vi "Parameter Druckregler.vi"(0 "Regelparameter":sgl[][](array[numeric]), 1 "Werte PMA":sgl[](array[numeric]), 2 "Werte FT-IR":sgl[](array[numeric]), 3 "Werte Ausgang":sgl[](array[numeric]), 4 "Werte NDIR":sgl[](array[numeric]), 5 "Werte Durchfluss":sgl[](array[numeric]), 6 "Werte Gaskühler":sgl[](array[numeric]), 7 "Werte Filterblock":sgl[](array[numeric]), 8 "Werte Kalter Block":sgl[](array[numeric]), 9 "Aktionen":T1) -> (10 "Werte Kalter Block":sgl[](array[numeric]), 12 "Werte Gaskühler":sgl[](array[numeric]), 13 "Werte Filterblock":sgl[](array[numeric]), 14 "Regleparameter":sgl[][](array[numeric]), 15 "Werte PMA":sgl[](array[numeric]), 16 "Werte FT-IR":sgl[](array[numeric]), 17 "Werte Ausgang":sgl[](array[numeric]), 18 "Werte NDIR":sgl[](array[numeric]), 19 "Werte Durchfluss":sgl[](array[numeric]))   [LabVIEW 2020, in "Regler.lvlib" / "Druckregler.lvlib"]
uses:
  Druckregler.lvlib
  Aktionen Param. Druckregler.ctl
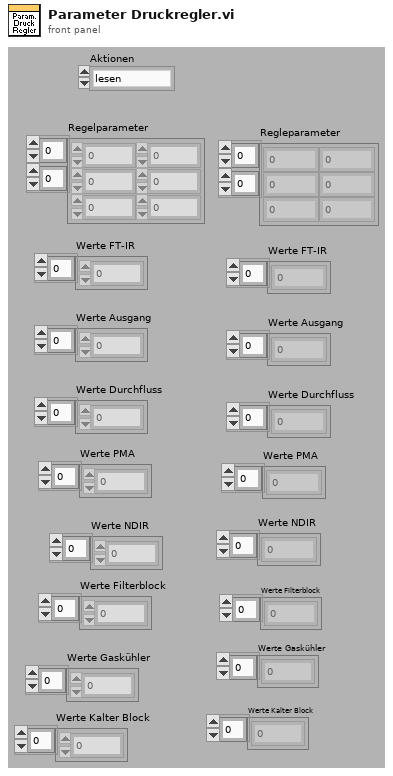
[diagram p1: front panel]
types:
  T1 = typedef "Regler.lvlib/Druckregler.lvlib/Aktionen Param. Druckregler.ctl" = enum16{"lesen", "schreiben", "Regler FT-IR", "Regler Ausgang", "Regler Durchfluss", "Regler PMA", "Regler NDIR", "Regler Filterblock", "Regler Gaskühler", "Regler Kalter Block"}
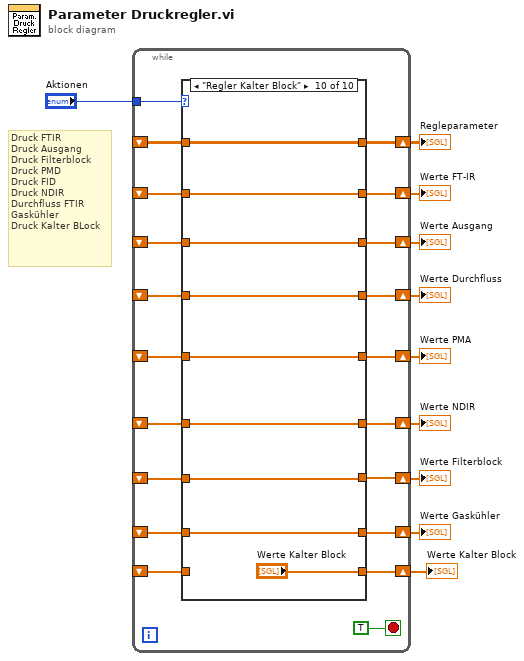
[diagram p0: block diagram]
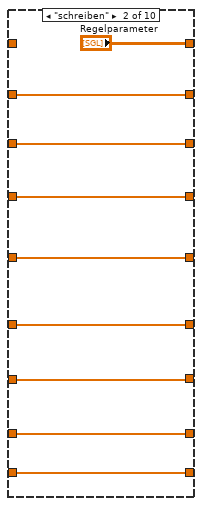
[diagram p3: hidden frame]
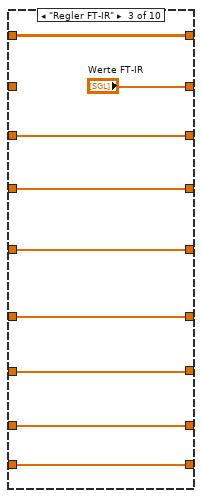
[diagram p4: hidden frame]
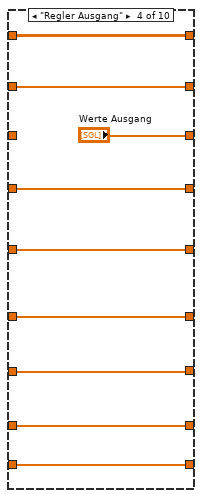
[diagram p5: hidden frame]
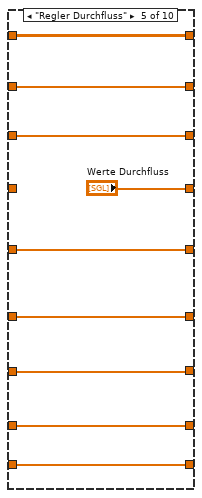
[diagram p6: hidden frame]
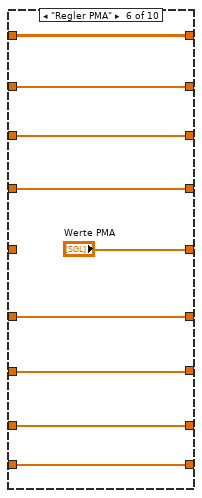
[diagram p7: hidden frame]
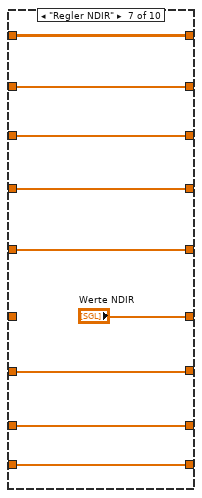
[diagram p8: hidden frame]
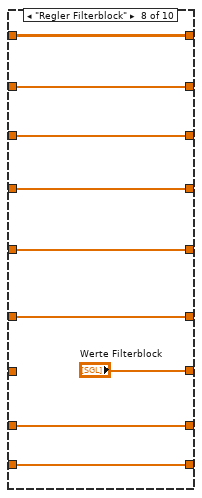
[diagram p9: hidden frame]
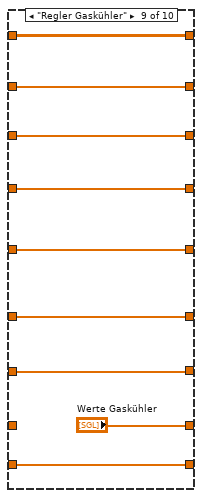
[diagram p10: hidden frame]
diagram:
  # "Druck FTIR\nDruck Ausgang\nDruck Filterblock\nDruck PMD\nDruck FID\nDruck NDIR\nDurchfluss FTIR\nGaskühler\nDruck Kalter BLock"
  n1 = while {
    tunnel: "Aktionen" -> [w29]
    shift-right: [w28] -> w9
    shift-left: _ -> [w27]
    shift-right: [w25] -> w8
    shift-left: _ -> [w26]
    shift-right: [w23] -> w7
    shift-left: _ -> [w24]
    shift-right: [w22] -> w6
    shift-left: _ -> [w21]
    shift-right: [w19] -> w5
    shift-left: _ -> [w20]
    shift-right: [w18] -> w4
    shift-left: _ -> [w17]
    shift-right: [w16] -> w3
    shift-left: _ -> [w15]
    shift-right: [w14] -> w2
    shift-left: _ -> [w13]
    shift-right: [w12] -> w1
    shift-left: _ -> [w11]
    stop <- TRUE stop-if-true
    n2 = case shown="\"Regler Kalter Block\"" w29 {
      tunnel: [w39 "Regelparameter" w56 w66 w72 w84 w93 w100 w111 w120] -> w28
      tunnel: w27 -> [w39 _ w56 w66 w72 w84 w93 w100 w111 w120]
      tunnel: w26 -> [w38 w47 _ w65 w73 w83 w92 w99 w110 w119]
      tunnel: [w38 w47 "Werte FT-IR" w65 w73 w83 w92 w99 w110 w119] -> w25
      tunnel: w24 -> [w37 w46 w55 _ w74 w82 w91 w98 w109 w118]
      tunnel: [w37 w46 w55 "Werte Ausgang" w74 w82 w91 w98 w109 w118] -> w23
      tunnel: [w36 w45 w54 w63 "Werte Durchfluss" w81 w90 w97 w108 w117] -> w22
      tunnel: w21 -> [w36 w45 w54 w63 _ w81 w90 w97 w108 w117]
      tunnel: w20 -> [w35 w44 w53 w62 w71 _ w89 w102 w107 w116]
      tunnel: [w35 w44 w53 w62 w71 "Werte PMA" w89 w102 w107 w116] -> w19
      tunnel: [w34 w43 w52 w61 w70 w79 "Werte NDIR" w101 w106 w115] -> w18
      tunnel: w17 -> [w34 w43 w52 w61 w70 w79 _ w101 w106 w115]
      tunnel: [w33 w42 w51 w60 w69 w78 w87 "Werte Filterblock" w105 w114] -> w16
      tunnel: w15 -> [w33 w42 w51 w60 w69 w78 w87 _ w105 w114]
      tunnel: [w32 w41 w50 w59 w68 w77 w86 w95 "Werte Gaskühler" w113] -> w14
      tunnel: w13 -> [w32 w41 w50 w59 w68 w77 w86 w95 _ w113]
      tunnel: [w31 w40 w49 w58 w67 w76 w85 w94 w103 "Werte Kalter Block"] -> w12
      tunnel: w11 -> [w31 w40 w49 w58 w67 w76 w85 w94 w103 _]
      frame "lesen", Default {
      }
      frame "schreiben" {
      }
      frame "Regler FT-IR" {
      }
      frame "Regler Ausgang" {
      }
      frame "Regler Durchfluss" {
      }
      frame "Regler PMA" {
      }
      frame "Regler NDIR" {
      }
      frame "Regler Filterblock" {
      }
      frame "Regler Gaskühler" {
      }
      frame "Regler Kalter Block" {
      }
    }
  }
  "Regleparameter" <- w9
  "Werte FT-IR" <- w8
  "Werte Ausgang" <- w7
  "Werte Durchfluss" <- w6
  "Werte PMA" <- w5
  "Werte NDIR" <- w4
  "Werte Filterblock" <- w3
  "Werte Gaskühler" <- w2
  "Werte Kalter Block" <- w1
